vi "CalcTotalScanCts.vi"(10 "Number of scan lines":i32, 11 "Motion Settings In":T1={"No Motion?"=FALSE, "Motion System"=enum."MM3000", "Motion Bd ID"=0, "Motion Profile"="SMAC1", "# Axis"=0, "Reverse Z axis?"=FALSE, "SMAC Axis"=0, "scan pair"=enum."y-(x) scan", "RT fps"=0.0, "Steps per mm"=[], "Motor Parameters"={"velocity ct/s"=[], "accel ct/s^2"=[]}, "One Way Scan"=FALSE, "Reverse One Way Scan"=FALSE, "Global Position (mm)"=[], "Plane"=0, "Distance between\nscan lines (um)"=0.0, "Distance between\nscan planes (um)"=0.0, "number of scan planes"=0, "Total steps in line"=0, "Xtra plane\ndistance  (um)"=0, "Xtra planes "=0, "Add Axis"=FALSE, "overshoot cts"=0, "BKPT Shift"=0, "Scan Start Time (ms)"=0, "ESP VISA"="", "3rd Axis"=1, "GL Ref Out"=refnum, "Galil Address"=""} {"3rd Axis" items=["x", "y", "z", "w"]; "Xtra planes" min=1; "Xtra plane\ndistance  (um)" min=0; "Distance between\nscan planes (um)" format="%.2f"; "Distance between\nscan lines (um)" format="%.2f"; "SMAC Axis" items=["None"=0, "Axis 1"=1, "Axis 2"=2, "Axis 3"=3, "Axis 4"=4, "Axis 5"=5, "Axis 6"=6, "Axis 7"=7, "Axis 8"=8, "Vector Space 1"=17, "Vector Space 2"=18, "Vector Space 3"=19, "Vector Space 4"=20]; "Motion Bd ID" min=1 max=32 step=1}) -> (3 "Total Steps":dbl)   [LabVIEW 2022 SP3]
uses:
  NI_controller/-NI_MotionRoutines/MotionParameters.ctl
  NI_controller/-NI_MotionRoutines/MotionSys.ctl
  ScanAxis.ctl
  3rdAxis.ctl
panel:
  # "1-D and 2-D B scan settings"
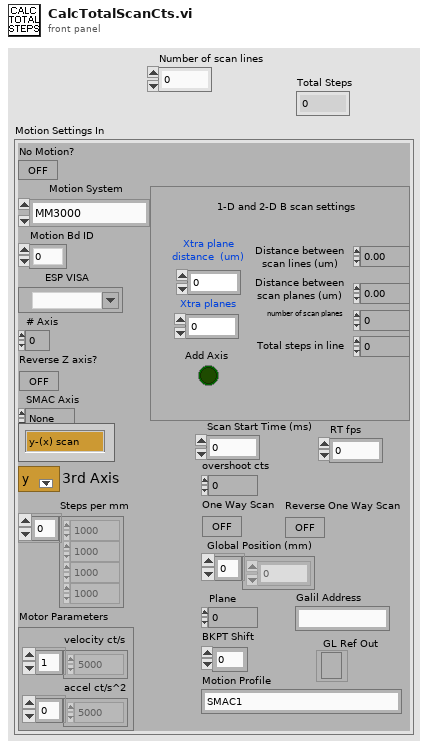
[diagram p1: front panel]
types:
  T1 = typedef "MotionParameters.ctl" = cluster{"No Motion?":bool, "Motion System":T2, "Motion Bd ID":u8, "Motion Profile":string, "# Axis":i8, "Reverse Z axis?":bool, "SMAC Axis":u16, "scan pair":T3, "RT fps":sgl, "Steps per mm":i32[], "Motor Parameters":cluster{"velocity ct/s":dbl[], "accel ct/s^2":dbl[]}, "One Way Scan":bool, "Reverse One Way Scan":bool, "Global Position (mm)":dbl[], "Plane":i32, "Distance between\nscan lines (um)":sgl, "Distance between\nscan planes (um)":sgl, "number of scan planes":i32, "Total steps in line":i32, "Xtra plane\ndistance  (um)":i32, "Xtra planes ":i32, "Add Axis":bool, "overshoot cts":i32, "BKPT Shift":i32, "Scan Start Time (ms)":u32, "ESP VISA":refnum<visa-resource-name>, "3rd Axis":T4, "GL Ref Out":refnum<k7>, "Galil Address":string}
  T2 = typedef "MotionSys.ctl" = enum16{"MM3000", "NI 735x", "Newport ESP", "No Motion Card", "Galil"}
  T3 = typedef "ScanAxis.ctl" = enum16{"y-(x) scan", "x-(y) scan", "z-(x) scan", "z-(y) scan", "y-(z) scan", "x-(z) scan", "w-(x) scan", "w-(y) scan", "w-(z) scan", "x-(w) scan", "y-(w) scan", "z-(w) scan"}
  T4 = typedef "3rdAxis.ctl" = u16
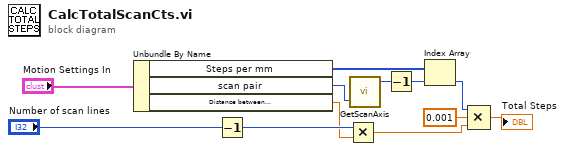
[diagram p0: block diagram]
diagram:
  n1 = Unbundle By Name("Motion Settings In") -> ("Steps per mm"=w10:i32[], "scan pair"=w4:T3, "Distance between\nscan lines (um)"=w3:sgl)
  n2 = Decrement(x="Number of scan lines") -> (x-1=w5:i32)
  n3 = Multiply(x=w5, y=w3) -> (x*y=w2:sgl)
  n4 = call "GetScanAxis.vi"("scan pair"=w4) -> ("Axis 1"=w11:i32)  [unwired: 1 in, 2 out]
  n5 = Decrement(x=w11) -> (x-1=w7:i32)
  n6 = Index Array(array=w10, index=w7) -> (element=w8:i32)
  n7 = Compound Arithmetic op=MULTIPLY(w8, 0.001, w2) -> (→"Total Steps":dbl)
